vi "Test Epochs (v1.2).vi"() -> ()   [LabVIEW 2017]
uses:
  source/epoch.UTC/Epoch.UTC.lvclass
  C:/Users/patrick/Documents/GitHub/Epoch-Time/source/epoch/Epoch.lvclass
  source/epoch/Epoch.lvclass
  source/epoch.GPS/Epoch.GPS.lvclass
  source/formatter.iso8601/DateTime.ISO8601.lvclass
  C:/Users/patrick/Documents/GitHub/Epoch-Time/source/formatter/DateTimeFormatter.lvclass
  source/formatter.iso8601/ISO8601 Date Formats.ctl
  source/Timestamp Compare Units -- enum.ctl
  source/epoch.UNIX/Epoch.UNIX.lvclass
  source/formatter.iso8601/DateTime.ISO8601.lvclass/DateTime.ISO8601.ctl
  source/isLeapYear (integer).vi
  source/isLeapYear (timestamp).vi
  source/formatter/DateTimeFormatter.lvclass
panel:
  out "RFC5322 Strict":bool
  out "RFC5322 UT":bool
  out "RFC5322 GMT":bool
  out "RFC5322 +0000":bool
  out "DST ISO8601":bool
  out "DST RFC5322":bool
  out "Merge-Split fractional seconds":bool
  out "(Split) Unix Time (s) from (us)":i64
  out "(Split) Fractional Second from (us)":dbl format="%#.6f"
  out "(Split) Unix Time (s) from (ms)":i64
  out "(Split) Fractional Second from (ms)":dbl format="%#.6f"
  out "(Split) Unix Time (s)":i64
  out "(Split) Fractional Second":dbl format="%#.6f"
  out "(Integer) Unix Time (us)":i64
  out "(Integer) Unix Time (ms)":i64
  out "(Float) Unix Time":dbl format="%#.6f"
  in  "Timestamp":timestamp
  out "Valid RFC3339 Dates":bool
  out "Valid ISO Dates":bool
  out "ISO Week":bool
  out "ISO DateTime (with UTC)":bool
  out "ISO DateTime (no UTC)":bool
  out "Ordinal Date Test":bool[](array[boolean])
  out "is Leap Year?":bool
  out "Weekday Test Vectors":bool[](array[boolean])
  out "ISO8601 DateTime (Week)":string
  out "Not a Timestamp?":bool
  out "ISO8601 DateTime (UTC)":string
  out "ISO8601 DateTime":string
  out "Local = Current Timestamp":bool
  out "Unix Time (s)":i64
  out "Unix = Local":bool
  out "GPS = Local Timestamp":bool
  out "GPS Time (s)":i64
  out "UTC = Local":bool
  out "current system time":timestamp
  out "UTC Time (s)":i64
  out "Fractional Second":dbl format="%#.6f"
  out "Local Time (s)":i64
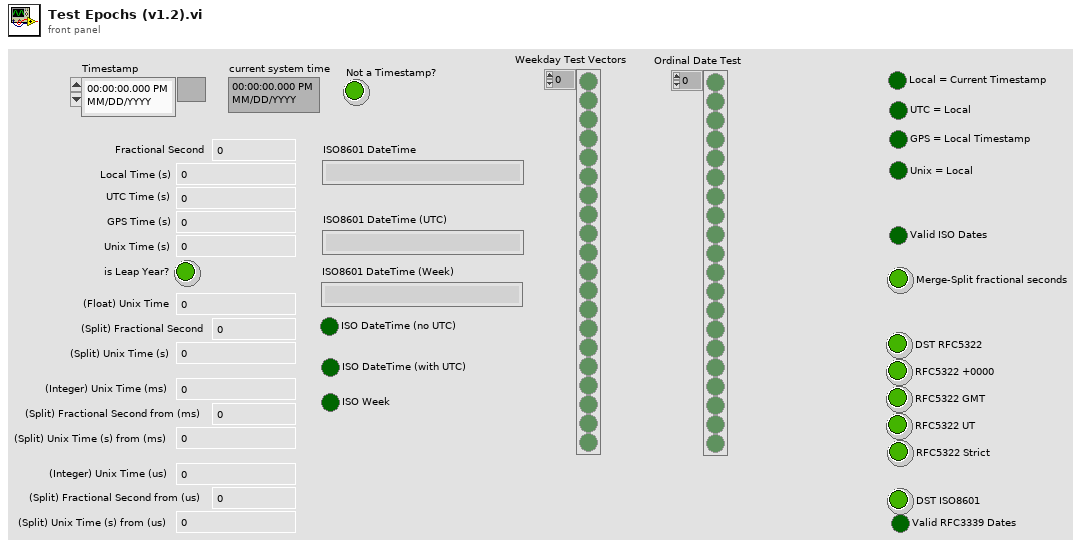
[diagram p1: front panel]
types:
  T1 = typedef "Timestamp Compare Units -- enum.ctl" = enum16{"week", "day", "hour", "minute", "second", "millisecond", "microsecond", "nanosecond"}
  T2 = typedef "ISO8601 Date Formats.ctl" = enum16{"UTC Date-Time", "ISO Time", "Date", "Calendar Month", "Week", "Week-Day", "Month-Day", "Ordinal Date"}
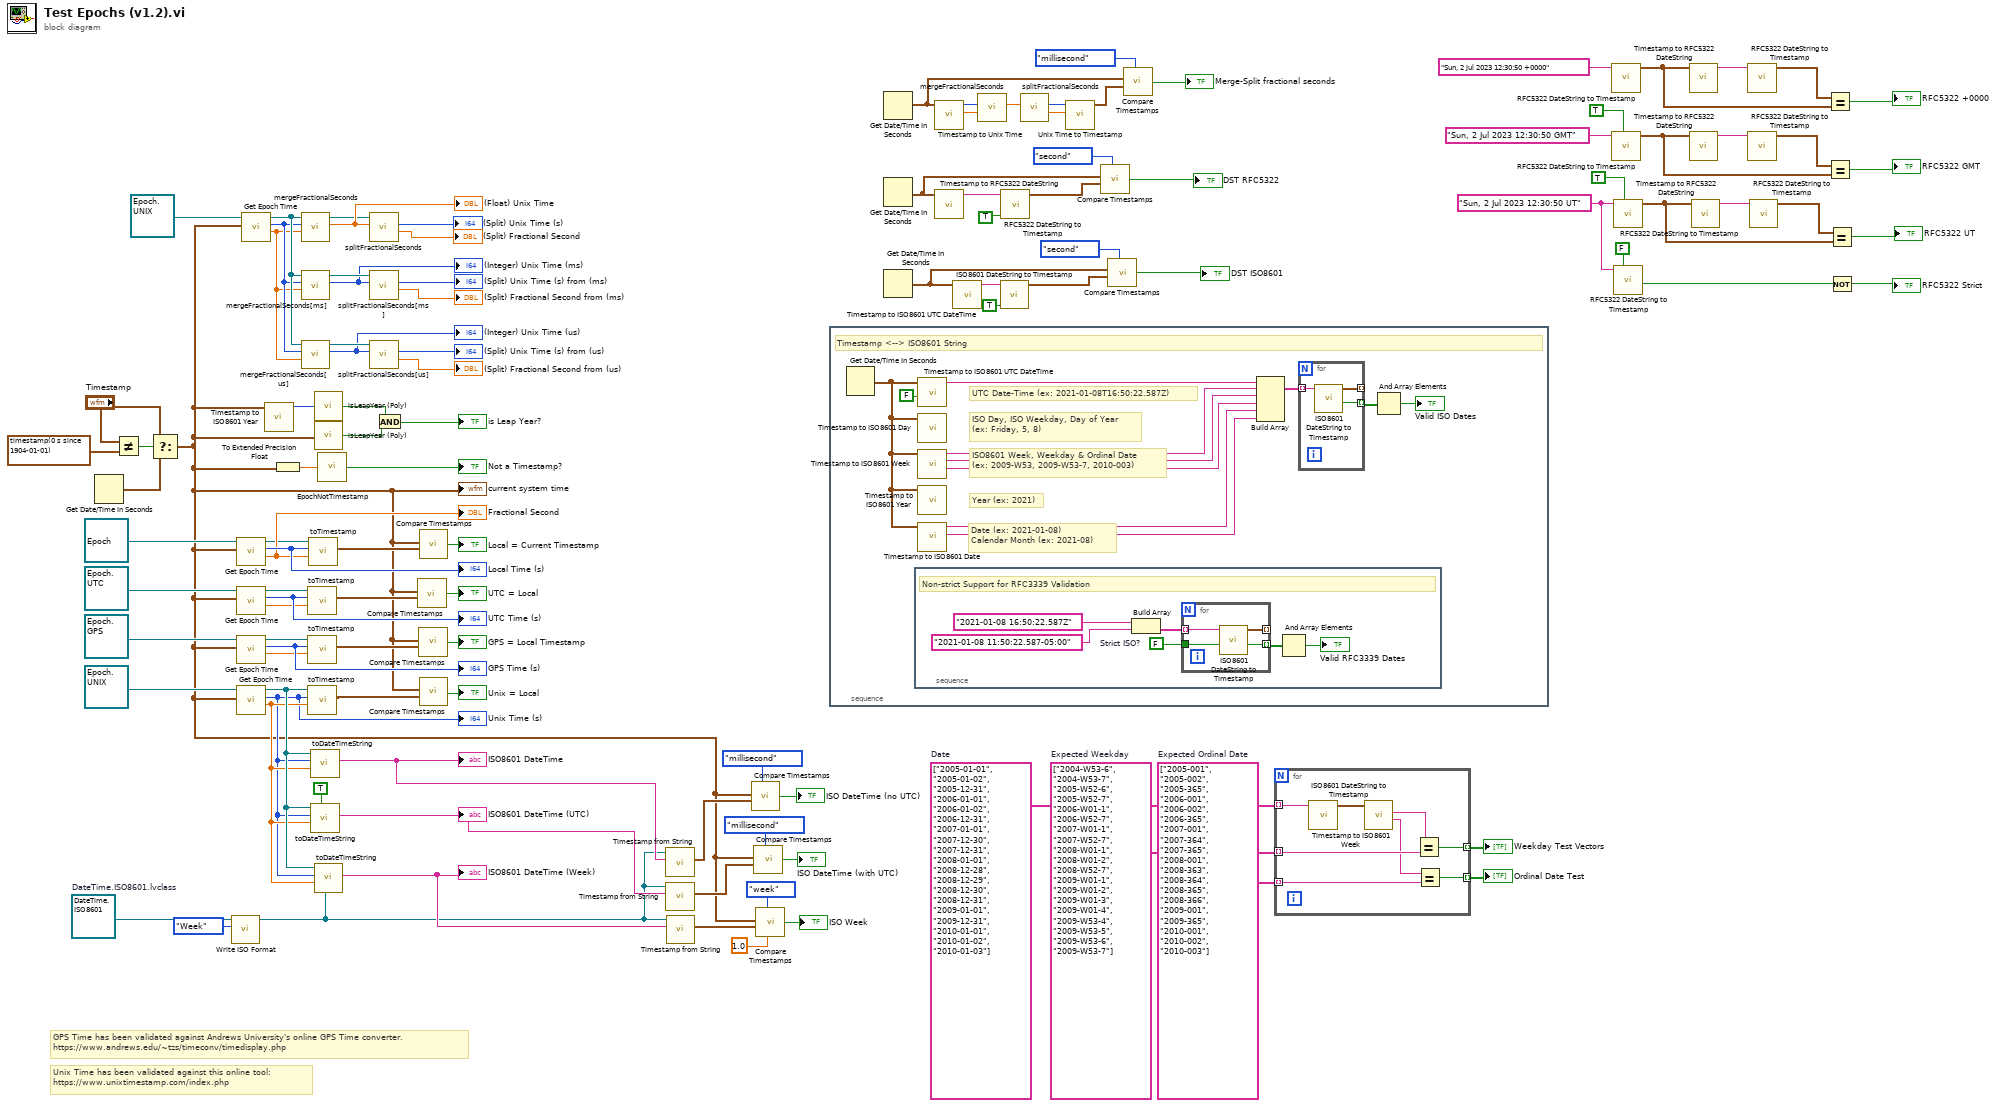
[diagram p0: block diagram]
diagram:
  w3 = "Sun, 2 Jul 2023 12:30:50 UT" ("RFC5322 Date String")
  w60 = string[] ["2005-01-01", "2005-01-02", "2005-12-31", "2006-01-01", "2006-01-02", "2006-12-31", "2007-01-01", "2007-12-30", "2007-12-31", "2008-01-01", "2008-12-28", "2008-12-29", "2008-12-30", "2008-12-31", "2009-01-01", "2009-12-31", "2010-01-01", "2010-01-02", "2010-01-03"]  # Date
  w91 = string[] ["2005-001", "2005-002", "2005-365", "2006-001", "2006-002", "2006-365", "2007-001", "2007-364", "2007-365", "2008-001", "2008-363", "2008-364", "2008-365", "2008-366", "2009-001", "2009-365", "2010-001", "2010-002", "2010-003"]  # Expected Ordinal Date
  w93 = string[] ["2004-W53-6", "2004-W53-7", "2005-W52-6", "2005-W52-7", "2006-W01-1", "2006-W52-7", "2007-W01-1", "2007-W52-7", "2008-W01-1", "2008-W01-2", "2008-W52-7", "2009-W01-1", "2009-W01-2", "2009-W01-3", "2009-W01-4", "2009-W53-4", "2009-W53-5", "2009-W53-6", "2009-W53-7"]  # Expected Weekday
  w94 = refnum<class "DateTime.ISO8601.lvclass"> refnum  # DateTime.ISO8601.lvclass
  # "Unix Time has been validated against this online tool:\nhttps://www.unixtimestamp.com/index.php"
  # "GPS Time has been validated against Andrews University's online GPS Time converter.\nhttps://www.andrews.edu/~tzs/timeconv/timedisplay.php"
  n1 = Get Date/Time In Seconds() -> (seconds since 1Jan1904=w69:timestamp)
  n2 = Not Equal?(x="Timestamp", y=timestamp(0 s since 1904-01-01)) -> (x != y?=w71:bool)
  n3 = Select(t="Timestamp", s=w71, f=w69) -> (s? t:f=w58:timestamp)
  "current system time" <- w58
  n4 = call "Write ISO Format.vi"("ISO Format"=ISO8601_Date_Formats."Week", "DateTime.ISO8601 in"=w94) -> ("DateTime.ISO8601 out"=w72:refnum<class "DateTime.ISO8601.lvclass">)  [unwired: 9 in]
  n5 = call "Get Epoch Time.vi"("Timestamp (now)"=w58, "Epoch (Local)"=refnum<class "Epoch.lvclass"> refnum ("Epoch.lvclass")) -> ("Fractional Second"=w106:dbl, "Epoch Time (s)"=w111:i64, "Epoch out"=w105:refnum<class "Epoch.lvclass">)  [unwired: 7 in]
  "Local Time (s)" <- w111
  "Fractional Second" <- w106
  n6 = call "Get Epoch Time.vi"("Timestamp (now)"=w58, "Epoch (Local)"=refnum<class "Epoch.UTC.lvclass"> refnum ("Epoch.UTC.lvclass")) -> ("Fractional Second"=w107:dbl, "Epoch Time (s)"=w112:i64, "Epoch out"=w108:refnum<class "Epoch.UTC.lvclass">)  [unwired: 7 in]
  "UTC Time (s)" <- w112
  n7 = call "Get Epoch Time.vi"("Timestamp (now)"=w58, "Epoch (Local)"=refnum<class "Epoch.GPS.lvclass"> refnum ("Epoch.GPS.lvclass")) -> ("Fractional Second"=w103:dbl, "Epoch Time (s)"=w109:i64, "Epoch out"=w102:refnum<class "Epoch.GPS.lvclass">)  [unwired: 7 in]
  "GPS Time (s)" <- w109
  n8 = call "Get Epoch Time.vi"("Timestamp (now)"=w58, "Epoch (Local)"=refnum<class "Epoch.UNIX.lvclass"> refnum ("Epoch.UNIX.lvclass")) -> ("Fractional Second"=w97:dbl, "Epoch Time (s)"=w95:i64, "Epoch out"=w98:refnum<class "Epoch.UNIX.lvclass">)  [unwired: 7 in]
  "Unix Time (s)" <- w95
  n9 = call "Get Epoch Time.vi"("Timestamp (now)"=w58, "Epoch (Local)"=refnum<class "Epoch.UNIX.lvclass"> refnum ("Epoch.UNIX.lvclass")) -> ("Fractional Second"=w54:dbl, "Epoch Time (s)"=w55:i64, "Epoch out"=w56:refnum<class "Epoch.UNIX.lvclass">)  [unwired: 7 in]
  n10 = call "Timestamp to ISO8601 Year.vi"("Timestamp (now)"=w58) -> ("year"=w89:i32)  [unwired: 9 in, 1 out]
  n11 = To Extended Precision Float(1:w58) -> (0:w100:ext)
  n12 = call "mergeFractionalSeconds.vi"("Fractional Second"=w54, "(Integer) Time (s)"=w55, "Epoch in"=w56) -> ("(Float) Time (s)"=w53:dbl, "Epoch out"=w52:refnum<class "Epoch.UNIX.lvclass">)  [unwired: 7 in]
  "(Float) Unix Time" <- w53
  n13 = call "mergeFractionalSeconds[ms].vi"("Fractional Second"=w54, "(Integer) Time (s)"=w55, "Epoch in"=w56) -> ("(Integer) Time (ms)"=w48:i64, "Epoch out"=w49:refnum<class "Epoch.UNIX.lvclass">)  [unwired: 7 in]
  "(Integer) Unix Time (ms)" <- w48
  n14 = call "mergeFractionalSeconds[us].vi"("Fractional Second"=w54, "(Integer) Time (s)"=w55, "Epoch in"=w56) -> ("(Integer) Time (us)"=w44:i64, "Epoch out"=w45:refnum<class "Epoch.UNIX.lvclass">)  [unwired: 7 in]
  "(Integer) Unix Time (us)" <- w44
  n15 = call-dynamic "toTimestamp.vi"("Fractional Second"=w107, "UTC Time (s)"=w112, "Epoch (UTC)"=w108) -> ("Timestamp"=w65:timestamp)  [unwired: 6 in, 2 out]
  n16 = call-dynamic "toTimestamp.vi"("Fractional Second"=w103, "GPS Time (s)"=w109, "Epoch (GPS)"=w102) -> ("Timestamp"=w61:timestamp)  [unwired: 6 in, 2 out]
  n17 = call-dynamic "toTimestamp.vi"("Fractional Second"=w97, "Unix Time (s)"=w95, "Epoch (Unix)"=w98) -> ("Timestamp"=w62:timestamp)  [unwired: 6 in, 2 out]
  n18 = call-dynamic "toTimestamp.vi"("Fractional Second"=w106, "Epoch Time (s)"=w111, "Epoch (Local)"=w105) -> ("Timestamp"=w66:timestamp)  [unwired: 6 in, 2 out]
  n19 = call "toDateTimeString.vi"("Fractional Second"=w97, "Epoch Time (s)"=w95, "Epoch"=w98) -> ("DateTime string"=w88:string)  [unwired: 6 in, 2 out]
  "ISO8601 DateTime" <- w88
  n20 = call "toDateTimeString.vi"("UTC? (F)"=TRUE, "Fractional Second"=w97, "Epoch Time (s)"=w95, "Epoch"=w98) -> ("DateTime string"=w87:string)  [unwired: 5 in, 2 out]
  "ISO8601 DateTime (UTC)" <- w87
  n21 = call-poly "isLeapYear (Poly).vi"("Year (0: this year)"=w89) -> ("is Leap Year?"=w85:bool)  [unwired: 8 in]
  n22 = call-poly "isLeapYear (Poly).vi"("timestamp (now)"=w58) -> ("is Leap Year?"=w84:bool)  [unwired: 8 in]
  n23 = call "toDateTimeString.vi"("DateTimeFormatter (ISO8601)"=w72, "Fractional Second"=w97, "Epoch Time (s)"=w95, "Epoch"=w98) -> ("DateTime string"=w86:string)  [unwired: 5 in, 2 out]
  "ISO8601 DateTime (Week)" <- w86
  n24 = call "EpochNotTimestamp.vi"("Epoch Time"=w100) -> ("Not a Timestamp?"=→"Not a Timestamp?":bool)  [unwired: 8 in]
  n25 = call "splitFractionalSeconds.vi"("(Float) Time (s)"=w53, "Epoch in"=w52) -> ("Fractional Second"=→"(Split) Fractional Second":dbl, "(Integer) Time (s)"=→"(Split) Unix Time (s)":i64)  [unwired: 7 in, 1 out]
  n26 = call "splitFractionalSeconds[ms].vi"("(Integer) Time (ms)"=w48, "Epoch in"=w49) -> ("Fractional Second"=→"(Split) Fractional Second from (ms)":dbl, "(Integer) Time (s)"=→"(Split) Unix Time (s) from (ms)":i64)  [unwired: 7 in, 1 out]
  n27 = call "splitFractionalSeconds[us].vi"("(Integer) Time (us)"=w44, "Epoch in"=w45) -> ("Fractional Second"=→"(Split) Fractional Second from (us)":dbl, "(Integer) Time (s)"=→"(Split) Unix Time (s) from (us)":i64)  [unwired: 7 in, 1 out]
  n28 = And(x=w85, y=w84) -> (x .and. y?=→"is Leap Year?":bool)
  n29 = call "Compare Timestamps.vi"("timestamp (1)"=w58, "timestamp (2)"=w65) -> ("Equal?"=→"UTC = Local":bool)  [unwired: 6 in]
  n30 = call "Compare Timestamps.vi"("timestamp (1)"=w58, "timestamp (2)"=w61) -> ("Equal?"=→"GPS = Local Timestamp":bool)  [unwired: 6 in]
  n31 = call "Compare Timestamps.vi"("timestamp (1)"=w58, "timestamp (2)"=w66) -> ("Equal?"=→"Local = Current Timestamp":bool)  [unwired: 6 in]
  n32 = call "Compare Timestamps.vi"("timestamp (1)"=w58, "timestamp (2)"=w62) -> ("Equal?"=→"Unix = Local":bool)  [unwired: 6 in]
  n33 = call "Timestamp from String.vi"("DateTime String"=w88, "DateTimeFormatter in"=w72) -> ("Timestamp"=w80:timestamp)  [unwired: 7 in, 2 out]
  n34 = call "Timestamp from String.vi"("DateTime String"=w87, "DateTimeFormatter in"=w72) -> ("Timestamp"=w79:timestamp)  [unwired: 7 in, 2 out]
  n35 = call "Timestamp from String.vi"("DateTime String"=w86, "DateTimeFormatter in"=w72) -> ("Timestamp"=w77:timestamp)  [unwired: 7 in, 2 out]
  n36 = call "Compare Timestamps.vi"("Unit (ms)"=Timestamp_Compare_Units_--_enum."millisecond" ("Unit (second)"), "timestamp (1)"=w58, "timestamp (2)"=w80) -> ("Equal?"=→"ISO DateTime (no UTC)":bool)  [unwired: 5 in]
  n37 = call "Compare Timestamps.vi"("Unit (ms)"=Timestamp_Compare_Units_--_enum."millisecond" ("Unit (second)"), "timestamp (1)"=w58, "timestamp (2)"=w79) -> ("Equal?"=→"ISO DateTime (with UTC)":bool)  [unwired: 5 in]
  n38 = call "Compare Timestamps.vi"("Unit (ms)"=Timestamp_Compare_Units_--_enum."week" ("Unit (second)"), "timestamp (1)"=w58, "timestamp (2)"=w77, "Resolution (in selected unit)"=1.0) -> ("Equal?"=→"ISO Week":bool)  [unwired: 4 in]
  n39 = stacked-sequence {
    frame #0 {
      # "Date (ex: 2021-01-08)\nCalendar Month (ex: 2021-08)"
      # "Year (ex: 2021)"
      # "ISO8601 Week, Weekday & Ordinal Date\n(ex: 2009-W53, 2009-W53-7, 2010-003)"
      # "ISO Day, ISO Weekday, Day of Year\n(ex: Friday, 5, 8)"
      # "UTC Date-Time (ex: 2021-01-08T16:50:22.587Z)"
      # "Timestamp <--> ISO8601 String"
      n40 = Get Date/Time In Seconds() -> (seconds since 1Jan1904=w124:timestamp)
      n41 = stacked-sequence {
        frame #0 {
          w128 = FALSE  # Strict ISO?
          # "Non-strict Support for RFC3339 Validation"
          n42 = Build Array("2021-01-08 16:50:22.587Z" ("x"), "2021-01-08 11:50:22.587-05:00" ("x")) -> (w131:string[])
          n43 = for {
            tunnel: w131 -> [w135] mode=indexing
            tunnel: [w134] -> w130 mode=indexing
            tunnel: w128 -> [w133]
            tunnel: [w132] -> _ mode=indexing
            n44 = call "ISO8601 DateString to Timestamp.vi"("Strict ISO? (T)"=w133, "ISO8601 String"=w135) -> ("valid?"=w134:bool, "Timestamp"=w132:timestamp)  [unwired: 7 in, 1 out]
          }
          n45 = And Array Elements(Boolean array=w130) -> (logical AND=→"Valid RFC3339 Dates":bool)
        }
      }
      n46 = call "Timestamp to ISO8601 UTC DateTime.vi"("UTC? (F)"=FALSE, "Timestamp (now)"=w124) -> ("ISO8601 String"=w123:string)  [unwired: 9 in]
      n47 = call "Timestamp to ISO8601 Day.vi"("Timestamp (now)"=w124) -> ()  [unwired: 8 in, 3 out]
      n48 = call "Timestamp to ISO8601 Week.vi"("Timestamp (now)"=w124) -> ("ISO8601 Ordinal Date"=w120:string, "ISO8601 Weekday"=w121:string, "ISO8601 Week"=w122:string)  [unwired: 8 in]
      n49 = call "Timestamp to ISO8601 Year.vi"("Timestamp (now)"=w124) -> ()  [unwired: 9 in, 2 out]
      n50 = call "Timestamp to ISO8601 Date.vi"("Timestamp (now)"=w124) -> ("ISO8601 Calendar Month"=w118:string, "ISO8601 Date"=w119:string)  [unwired: 9 in]
      n51 = Build Array(w123, w122, w121, w120, w119, w118) -> (w117:string[])
      n52 = for {
        tunnel: w117 -> [w138] mode=indexing
        tunnel: [w137] -> w116 mode=indexing
        tunnel: [w136] -> _ mode=indexing
        n53 = call "ISO8601 DateString to Timestamp.vi"("ISO8601 String"=w138) -> ("valid?"=w137:bool, "Timestamp"=w136:timestamp)  [unwired: 8 in, 1 out]
      }
      n54 = And Array Elements(Boolean array=w116) -> (logical AND=→"Valid ISO Dates":bool)
    }
  }
  n55 = Get Date/Time In Seconds() -> (seconds since 1Jan1904=w35:timestamp)
  n56 = Get Date/Time In Seconds() -> (seconds since 1Jan1904=w29:timestamp)
  n57 = Get Date/Time In Seconds() -> (seconds since 1Jan1904=w25:timestamp)
  n58 = call "Timestamp to Unix Time.vi"("Timestamp (now)"=w35) -> ("Fractional Second"=w40:dbl, "Unix Time (s)"=w41:i64)  [unwired: 9 in]
  n59 = call "Timestamp to RFC5322 DateString.vi"("Timestamp (now)"=w29) -> ("RFC5322 Date String"=w32:string)  [unwired: 10 in]
  n60 = call "Timestamp to ISO8601 UTC DateTime.vi"("Timestamp (now)"=w25) -> ("ISO8601 String"=w24:string)  [unwired: 10 in]
  n61 = call "mergeFractionalSeconds.vi"("Fractional Second"=w40, "(Integer) Time (s)"=w41) -> ("(Float) Time (s)"=w39:dbl)  [unwired: 8 in, 1 out]
  n62 = call "ISO8601 DateString to Timestamp.vi"("deprecated"=TRUE ("Adjust for Local DST? (T)"), "ISO8601 String"=w24) -> ("Timestamp"=w23:timestamp)  [unwired: 7 in, 2 out]
  n63 = call "RFC5322 DateString to Timestamp.vi"("deprecated"=TRUE ("Adjust for Local DST? (T)"), "RFC5322 String"=w32) -> ("Timestamp"=w30:timestamp)  [unwired: 7 in, 2 out]
  n64 = call "splitFractionalSeconds.vi"("(Float) Time (s)"=w39) -> ("Fractional Second"=w37:dbl, "(Integer) Time (s)"=w38:i64)  [unwired: 8 in, 1 out]
  n65 = call "Unix Time to Timestamp.vi"("Fractional Second"=w37, "Unix Time (s)"=w38) -> ("Timestamp"=w36:timestamp)  [unwired: 8 in, 1 out]
  n66 = call "Compare Timestamps.vi"("Unit (ms)"=Timestamp_Compare_Units_--_enum."second", "timestamp (1)"=w29, "timestamp (2)"=w30) -> ("Equal?"=→"DST RFC5322":bool)  [unwired: 5 in]
  n67 = call "Compare Timestamps.vi"("Unit (ms)"=Timestamp_Compare_Units_--_enum."second", "timestamp (1)"=w25, "timestamp (2)"=w23) -> ("Equal?"=→"DST ISO8601":bool)  [unwired: 5 in]
  n68 = call "Compare Timestamps.vi"("Unit (ms)"=Timestamp_Compare_Units_--_enum."millisecond", "timestamp (1)"=w35, "timestamp (2)"=w36) -> ("Equal?"=→"Merge-Split fractional seconds":bool)  [unwired: 5 in]
  n69 = for {
    tunnel: w93 -> [w145] mode=indexing
    tunnel: [w146] -> w92 mode=indexing
    tunnel: w91 -> [w144] mode=indexing
    tunnel: [w143] -> w90 mode=indexing
    tunnel: w60 -> [w140] mode=indexing
    n70 = call "ISO8601 DateString to Timestamp.vi"("ISO8601 String"=w140) -> ("Timestamp"=w139:timestamp)  [unwired: 8 in, 2 out]
    n71 = call "Timestamp to ISO8601 Week.vi"("Timestamp (now)"=w139) -> ("ISO8601 Ordinal Date"=w142:string, "ISO8601 Weekday"=w141:string)  [unwired: 8 in, 1 out]
    n72 = Equal?(x=w141, y=w145) -> (x = y?=w146:bool)
    n73 = Equal?(x=w142, y=w144) -> (x = y?=w143:bool)
  }
  "Weekday Test Vectors" <- w92
  "Ordinal Date Test" <- w90
  n74 = call "RFC5322 DateString to Timestamp.vi"("RFC5322 String"="Sun, 2 Jul 2023 12:30:50 +0000" ("RFC5322 Date String")) -> ("Timestamp"=w16:timestamp)  [unwired: 8 in, 2 out]
  n75 = call "RFC5322 DateString to Timestamp.vi"("RFC850|ANSI-C permissive?"=TRUE, "RFC5322 String"="Sun, 2 Jul 2023 12:30:50 GMT" ("RFC5322 Date String")) -> ("Timestamp"=w15:timestamp)  [unwired: 7 in, 2 out]
  n76 = call "RFC5322 DateString to Timestamp.vi"("RFC850|ANSI-C permissive?"=TRUE, "RFC5322 String"=w3) -> ("Timestamp"=w7:timestamp)  [unwired: 7 in, 2 out]
  n77 = call "RFC5322 DateString to Timestamp.vi"("RFC850|ANSI-C permissive?"=FALSE, "RFC5322 String"=w3) -> ("valid?"=w2:bool)  [unwired: 7 in, 2 out]
  n78 = call "Timestamp to RFC5322 DateString.vi"("Timestamp (now)"=w16) -> ("RFC5322 Date String"=w19:string)  [unwired: 10 in]
  n79 = call "Timestamp to RFC5322 DateString.vi"("Timestamp (now)"=w15) -> ("RFC5322 Date String"=w12:string)  [unwired: 10 in]
  n80 = call "Timestamp to RFC5322 DateString.vi"("Timestamp (now)"=w7) -> ("RFC5322 Date String"=w9:string)  [unwired: 10 in]
  n81 = call "RFC5322 DateString to Timestamp.vi"("RFC5322 String"=w19) -> ("Timestamp"=w17:timestamp)  [unwired: 8 in, 2 out]
  n82 = call "RFC5322 DateString to Timestamp.vi"("RFC5322 String"=w12) -> ("Timestamp"=w14:timestamp)  [unwired: 8 in, 2 out]
  n83 = call "RFC5322 DateString to Timestamp.vi"("RFC5322 String"=w9) -> ("Timestamp"=w8:timestamp)  [unwired: 8 in, 2 out]
  n84 = Equal?(x=w17, y=w16) -> (x = y?=→"RFC5322 +0000":bool)
  n85 = Equal?(x=w14, y=w15) -> (x = y?=→"RFC5322 GMT":bool)
  n86 = Equal?(x=w8, y=w7) -> (x = y?=→"RFC5322 UT":bool)
  n87 = Not(x=w2) -> (.not. x?=→"RFC5322 Strict":bool)
